vi "Post-Uninstall Custom Action.vi"(10 "Variant":variant) -> (0 "error out":errorcluster)   [LabVIEW 2019]
uses:
  <resource>/dialog/lvconfig.llb/LV Config Read String.vi
  <vilib>/Utility/config.llb/Read Key (String).vi
  <vilib>/Utility/config.llb/Read Key (I32).vi
  <resource>/dialog/lvconfig.llb/LV Config Write String.vi
  <resource>/dialog/lvconfig.llb/LV Config Write Numeric (I32).vi
  <vilib>/Utility/config.llb/NI_LVConfig.lvlib
  <vilib>/zip/NI_Unzip.lvlib
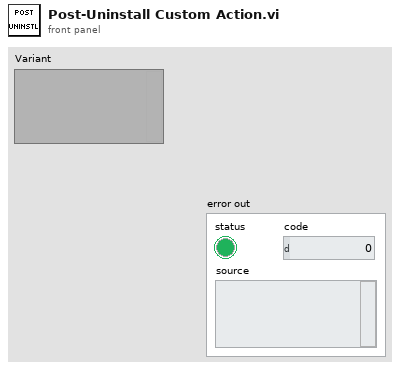
[diagram p1: front panel]
types:
  T1 = typedef "NI_LVConfig.lvlib/Config Data RefNum.ctl" = refnum<k1>
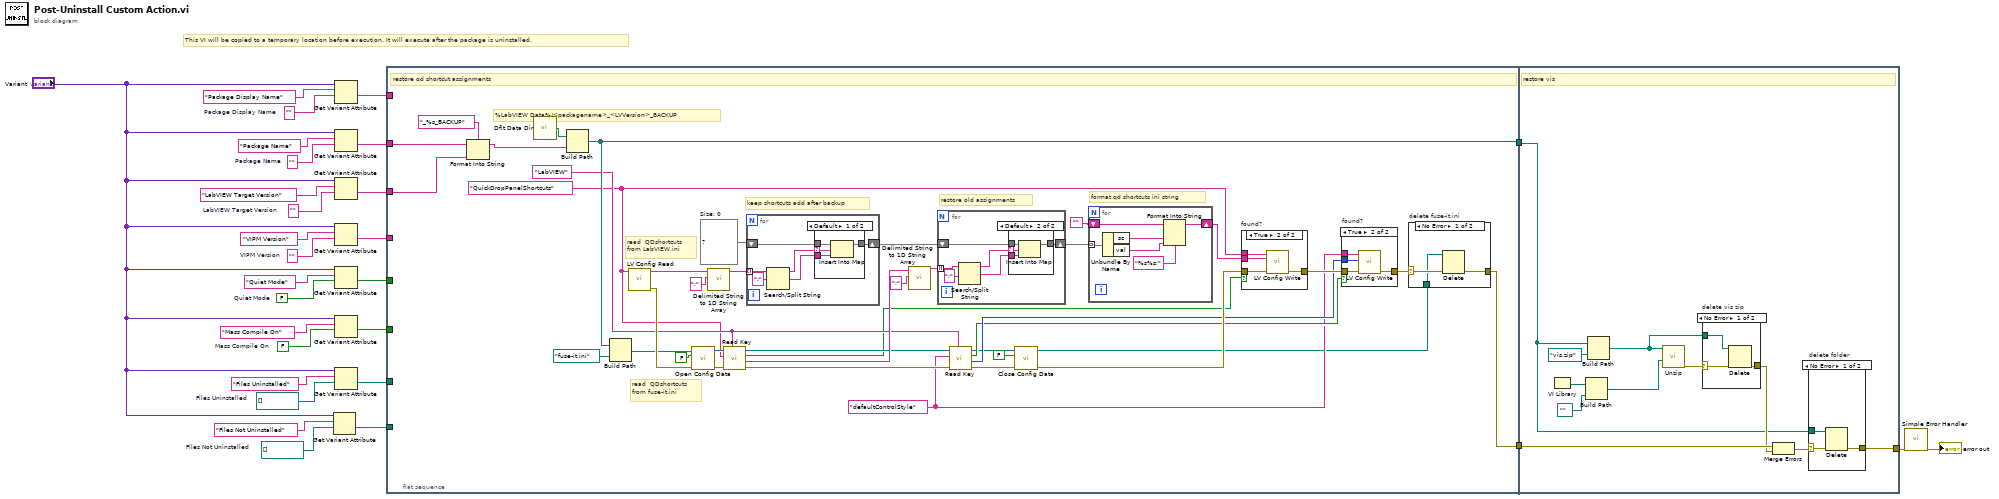
[diagram p0: block diagram]
diagram:
  w2 = path[] []  # Files Not Uninstalled
  w3 = path[] []  # Files Uninstalled
  w9 = FALSE  # Mass Compile On
  w10 = ""  # Package Display Name
  w17 = FALSE  # Quiet Mode
  w20 = ""  # VIPM Version
  w22 = ""  # LabVIEW Target Version
  w24 = ""  # Package Name
  # "This VI will be copied to a temporary location before execution. It will execute after the package is uninstalled."
  n1 = Get Variant Attribute(Variant="Variant", name="Files Not Uninstalled", default value (empty Variant)=w2) -> (value=w7:path[])  [unwired: 1 in, 3 out]
  n2 = Get Variant Attribute(Variant="Variant", name="Package Display Name", default value (empty Variant)=w10) -> (value=w16:string)  [unwired: 1 in, 3 out]
  n3 = Get Variant Attribute(Variant="Variant", name="Package Name", default value (empty Variant)=w24) -> (value=w15:string)  [unwired: 1 in, 3 out]
  n4 = Get Variant Attribute(Variant="Variant", name="LabVIEW Target Version", default value (empty Variant)=w22) -> (value=w14:string)  [unwired: 1 in, 3 out]
  n5 = Get Variant Attribute(Variant="Variant", name="VIPM Version", default value (empty Variant)=w20) -> (value=w13:string)  [unwired: 1 in, 3 out]
  n6 = Get Variant Attribute(Variant="Variant", name="Quiet Mode", default value (empty Variant)=w17) -> (value=w12:bool)  [unwired: 1 in, 3 out]
  n7 = Get Variant Attribute(Variant="Variant", name="Mass Compile On", default value (empty Variant)=w9) -> (value=w11:bool)  [unwired: 1 in, 3 out]
  n8 = Get Variant Attribute(Variant="Variant", name="Files Uninstalled", default value (empty Variant)=w3) -> (value=w6:path[])  [unwired: 1 in, 3 out]
  n9 = flat-sequence {
    tunnel: w16 -> [_]
    tunnel: w15 -> [w32]
    tunnel: w14 -> [w31]
    tunnel: w13 -> [_]
    tunnel: w12 -> [_]
    tunnel: w11 -> [_]
    tunnel: w6 -> [_]
    tunnel: w7 -> [_]
    tunnel: [w68] -> w28
    tunnel: [w55] -> w1
    tunnel: [w117] -> w29
    tunnel: w28 -> [w121]
    tunnel: w1 -> [w111]
    frame #0 {
      w50 = map{string, string} {}  # Size: 0
      w54 = "defaultControlStyle" ("key")
      w39 = "LabVIEW" ("section")
      w36 = "QuickDropPanelShortcuts" ("key")
      # "restore old assignments"
      # "format qd shortcuts ini string"
      # "read  QDshortcuts\nfrom fuse-it.ini"
      # "read  QDshortcuts\nfrom LabVIEW.ini"
      # "keep shortcuts add after backup"
      # "%LabVIEW Data%/<packagename>_<LVVersion>_BACKUP"
      # "restore qd shortcut assignments"
      n10 = Format Into String(format string="_%s_BACKUP", initial string=w32, w31) -> (resulting string=w30:string)  [unwired: 1 in, 1 out]
      n11 = call <vilib>:"Dflt Data Dir.vi"() -> ("App:Default Data Directory"=w60:path)
      n12 = Build Path(base path=w60, name or relative path=w30) -> (appended path=w55:path)
      n13 = Build Path(base path=w55, name or relative path=path "fuse-it.ini") -> (appended path=w38:path)
      n14 = call-poly <resource>:"LV Config Read.vi"("key"=w36) -> ("error out"=w65:errorcluster, "value"=w49:string)  [unwired: 4 in, 1 out]
      n15 = call <vilib>:"Open Config Data.vi"("error in (no error)"=w65, "create file if necessary (T)"=FALSE, "configuration file path"=w38) -> ("error out"=w66:errorcluster, "refnum"=w42:T1)  [unwired: 6 in, 1 out]
      n16 = call <vilib>:"Delimited String to 1D String Array.vi"("delimiter"=";", "delimited string"=w49) -> ("string array"=w51:string[])  [unwired: 9 in]
      n17 = call-poly <vilib>:"Read Key.vi"("section"=w39, "error in (no error)"=w66, "key"=w36, "refnum"=w42) -> ("error out"=w64:errorcluster, "value"=w41:string, "found?"=w34:bool, "refnum out"=w40:T1)  [unwired: 4 in]
      n18 = for {
        tunnel: w51 -> [w78] mode=indexing
        shift-right: [w76] -> w47
        shift-left: w50 -> [w77]
        n19 = Search/Split String(string=w78, search string/char (-)=":") -> (substring before match=w75:string, match + rest of string=w74:string)  [unwired: 1 in, 1 out]
        n20 = case shown="Default" w75 {
          selector: w75 -> [w81 _]
          tunnel: w77 -> [w83 w84]
          tunnel: [w82 w84] -> w76
          tunnel: w74 -> [w80 _]
          frame Default {
            n21 = Insert Into Map(map in=w83, key=w81, value=w80) -> (map out=w82:map{string, string})  [unwired: 2 out]
          }
          frame "" {
          }
        }
      }
      n22 = call <vilib>:"Delimited String to 1D String Array.vi"("delimiter"=";", "delimited string"=w41) -> ("string array"=w46:string[])  [unwired: 9 in]
      n23 = for {
        shift-right: [w90] -> w44
        shift-left: w47 -> [w89]
        tunnel: w46 -> [w87] mode=indexing
        n24 = Search/Split String(string=w87, search string/char (-)=":") -> (substring before match=w86:string, match + rest of string=w85:string)  [unwired: 1 in, 1 out]
        n25 = case shown="Default" w86 {
          selector: w86 -> [_ w93]
          tunnel: [w91 w95] -> w90
          tunnel: w89 -> [w91 w94]
          tunnel: w85 -> [_ w92]
          frame "" {
          }
          frame Default {
            n26 = Insert Into Map(map in=w94, key=w93, value=w92) -> (map out=w95:map{string, string})  [unwired: 2 out]
          }
        }
      }
      n27 = call-poly <vilib>:"Read Key.vi"("section"=w39, "error in (no error)"=w64, "key"=w54, "refnum"=w40) -> ("error out"=w67:errorcluster, "value"=w59:i32, "found?"=w58:bool, "refnum out"=w57:T1)  [unwired: 4 in]
      n28 = call <vilib>:"Close Config Data.vi"("error in (no error)"=w67, "write file if changed (T)"=FALSE, "refnum"=w57) -> ("error out"=w63:errorcluster, "file path"=w37:path)  [unwired: 7 in]
      n29 = for {
        tunnel: w44 -> [w101] mode=indexing
        shift-right: [w96] -> w35
        shift-left: "" -> [w99]
        n30 = Unbundle By Name(w101) -> ("sc"=w98:string, "val"=w97:string)
        n31 = Format Into String(format string="%s%s;", initial string=w99, w98, w97) -> (resulting string=w96:string)  [unwired: 1 in, 1 out]
      }
      n32 = case "found?" shown="True" w34 {
        tunnel: w36 -> [_ w71]
        tunnel: [w69 w72] -> w62
        tunnel: w63 -> [w69 w73]
        tunnel: w35 -> [_ w70]
        frame False {
        }
        frame True {
          n33 = call-poly <resource>:"LV Config Write.vi"("error in (no error)"=w73, "value"=w70, "key"=w71) -> ("error out"=w72:errorcluster)  [unwired: 4 in]
        }
      }
      n34 = case "found?" shown="True" w58 {
        tunnel: w62 -> [w102 w106]
        tunnel: [w102 w105] -> w61
        tunnel: w59 -> [_ w103]
        tunnel: w54 -> [_ w104]
        frame False {
        }
        frame True {
          n35 = call-poly <resource>:"LV Config Write.vi"("error in (no error)"=w106, "value"=w103, "key"=w104) -> ("error out"=w105:errorcluster)  [unwired: 4 in]
        }
      }
      n36 = case "delete fuse-it.ini" shown="No Error" w61 {
        selector: w61 -> [w109 w110]
        tunnel: w37 -> [w107 _]
        tunnel: [w108 w110] -> w68
        frame No Error {
          n37 = Delete(path (use dialog)=w107, error in=w109) -> (error out=w108:errorcluster)  [unwired: 3 in, 2 out]
        }
        frame Error {
        }
      }
    }
    frame #1 {
      # "restore vis"
      n38 = VI Library() -> (path=w114:path)
      n39 = Build Path(base path=w114, name or relative path=path "..") -> (appended path=w115:path)
      n40 = Build Path(base path=w111, name or relative path=path "vis.zip") -> (appended path=w112:path)
      n41 = call <vilib>:"Unzip.vi"("Target directory (same as Zip file if empty)"=w115, "Zip file"=w112) -> ("error out"=w120:errorcluster)  [unwired: 7 in, 2 out]
      n42 = case "delete vis zip" shown="No Error" w120 {
        selector: w120 -> [w124 w125]
        tunnel: w112 -> [w122 _]
        tunnel: [w123 w125] -> w119
        frame No Error {
          n43 = Delete(path (use dialog)=w122, error in=w124) -> (error out=w123:errorcluster)  [unwired: 3 in, 2 out]
        }
        frame Error {
        }
      }
      n44 = Merge Errors(w121, w119) -> (w118:errorcluster)
      n45 = case "delete folder" shown="No Error" w118 {
        selector: w118 -> [w128 w129]
        tunnel: w111 -> [w126 _]
        tunnel: [w127 w129] -> w117
        frame No Error {
          n46 = Delete(path (use dialog)=w126, error in=w128) -> (error out=w127:errorcluster)  [unwired: 3 in, 2 out]
        }
        frame Error {
        }
      }
    }
  }
  n47 = call <vilib>:"Simple Error Handler.vi"("error in (no error)"=w29) -> ("error out"=→"error out":errorcluster)  [unwired: 4 in, 4 out]
